vi "Get Attribute I32.vi"(8 "error in":errorcluster, 10 "Attribute":string, 11 "IConfiguration in":refnum<class "IConfiguration.lvclass">) -> (0 "error out":errorcluster, 2 "Value":i32, 3 "IConfiguration out":refnum<class "IConfiguration.lvclass">)   [LabVIEW 2024, in "IConfiguration.lvclass"]
uses:
  IConfiguration.lvclass
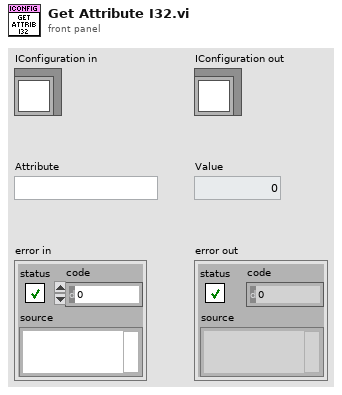
[diagram p1: front panel]
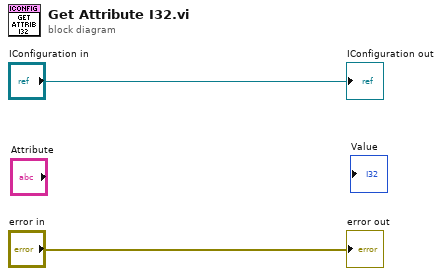
[diagram p0: block diagram]
diagram:
  "error out" <- "error in"
  "IConfiguration out" <- "IConfiguration in"
